vi "Is Device Connected.vi"(8 "error in (no error)":errorcluster, 10 "Serial Number":string="97000001") -> (0 "error out":errorcluster, 2 "Is Device Connected":bool)   [LabVIEW 2017, in "XYStage.KIM101.lvclass"]
uses:
  XYStage.KIM101.lvclass
  C:/Program Files (x86)/Thorlabs/Kinesis/Thorlabs.MotionControl.DeviceManagerCLI.dll
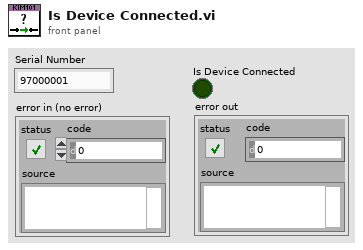
[diagram p1: front panel]
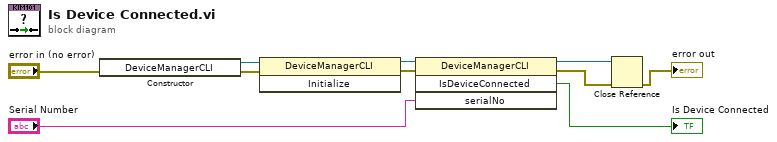
[diagram p0: block diagram]
diagram:
  n1 = constructor class="DeviceManagerCLI"(error in="error in (no error)") -> (reference out=w7:refnum<k24>, error out=w6:errorcluster)  [unwired: 2 in, 1 out]
  n2 = invoke class="DeviceManagerCLI" method="Initialize"(reference=w7, error in=w6) -> (reference out=w8:refnum<k24>, error out=w4:errorcluster)  [unwired: 1 in, 1 out]
  n3 = invoke class="DeviceManagerCLI" method="IsDeviceConnected"(reference=w8, error in=w4, "serialNo"="Serial Number") -> (reference out=w3:refnum<k24>, error out=w2:errorcluster, "IsDeviceConnected"=→"Is Device Connected":bool)  [unwired: 1 in, 1 out]
  n4 = Close Reference(reference=w3, error in (no error)=w2) -> (error out=→"error out":errorcluster)
